vi "CreateSwapArray_v4.vi"(8 "error in (no error)":errorcluster, 9 "ROSCO Params":T3, 11 "ArrayPairs":T1={"iStatus"={"Index"=0, "Value"=0.0}, "TIME"={"Index"=1, "Value"=0.0}, "DT"={"Index"=2, "Value"=0.0}, "BL_PITCH"={"Index"=3, "Value"=0.0}, "VS_MECHGENPWR"={"Index"=13, "Value"=0.0}, "VS_GENPWR"={"Index"=14, "Value"=0.0}, "GEN_SPEED"={"Index"=19, "Value"=0.0}, "ROTOR_SPEED"={"Index"=20, "Value"=0.0}, "GENTQMEAS"={"Index"=22, "Value"=0.0}, "Y_M"={"Index"=23, "Value"=0.0}, "HORWINDV"={"Index"=26, "Value"=0.0}, "ROOTMOOP1"={"Index"=29, "Value"=0.0}, "ROOTMOOP2"={"Index"=30, "Value"=0.0}, "BL_PITCH2"={"Index"=32, "Value"=0.0}, "BL_PITCH3"={"Index"=33, "Value"=0.0}, "ROOTMOOP3"={"Index"=31, "Value"=0.0}, "AVCMSG_SIZE"={"Index"=48, "Value"=0.0}, "INFILE_SIZE "={"Index"=49, "Value"=0.0}, "OUTFILE_SIZE "={"Index"=50, "Value"=0.0}, "FA_ACC"={"Index"=52, "Value"=0.0}, "NUM_BLADES"={"Index"=60, "Value"=0.0}, "OUT_BL_PITCH"={"Index"=44, "Value"=0.0}, "OUT_TORQUE"={"Index"=46, "Value"=0.0}, "OUT_AEROTQ"={"Index"=89, "Value"=0.0}, "Out.RotSpeed "={"Index"=92, "Value"=0.0}, "Out.DEBUG"={"Index"=93, "Value"=0.0}}) -> (0 "error out":errorcluster, 1 "ROSCO Params Out":T3, 3 "ArrayPairs Out":T1={"iStatus"={"Index"=0, "Value"=0.0}, "TIME"={"Index"=1, "Value"=0.0}, "DT"={"Index"=2, "Value"=0.0}, "BL_PITCH"={"Index"=3, "Value"=0.0}, "VS_MECHGENPWR"={"Index"=13, "Value"=0.0}, "VS_GENPWR"={"Index"=14, "Value"=0.0}, "GEN_SPEED"={"Index"=19, "Value"=0.0}, "ROTOR_SPEED"={"Index"=20, "Value"=0.0}, "GENTQMEAS"={"Index"=22, "Value"=0.0}, "Y_M"={"Index"=23, "Value"=0.0}, "HORWINDV"={"Index"=26, "Value"=0.0}, "ROOTMOOP1"={"Index"=29, "Value"=0.0}, "ROOTMOOP2"={"Index"=30, "Value"=0.0}, "BL_PITCH2"={"Index"=32, "Value"=0.0}, "BL_PITCH3"={"Index"=33, "Value"=0.0}, "ROOTMOOP3"={"Index"=31, "Value"=0.0}, "AVCMSG_SIZE"={"Index"=48, "Value"=0.0}, "INFILE_SIZE "={"Index"=49, "Value"=0.0}, "OUTFILE_SIZE "={"Index"=50, "Value"=0.0}, "FA_ACC"={"Index"=52, "Value"=0.0}, "NUM_BLADES"={"Index"=60, "Value"=0.0}, "OUT_BL_PITCH"={"Index"=44, "Value"=0.0}, "OUT_TORQUE"={"Index"=46, "Value"=0.0}, "OUT_AEROTQ"={"Index"=89, "Value"=0.0}, "Out.RotSpeed "={"Index"=92, "Value"=0.0}, "Out.DEBUG"={"Index"=93, "Value"=0.0}}, 4 "avrSWAP":sgl[](array[numeric]))   [LabVIEW 2018]
uses:
  Clusters/RoscoParams.ctl
  Clusters/ArrayPairs.ctl
  Clusters/SwapArrayCluster.ctl
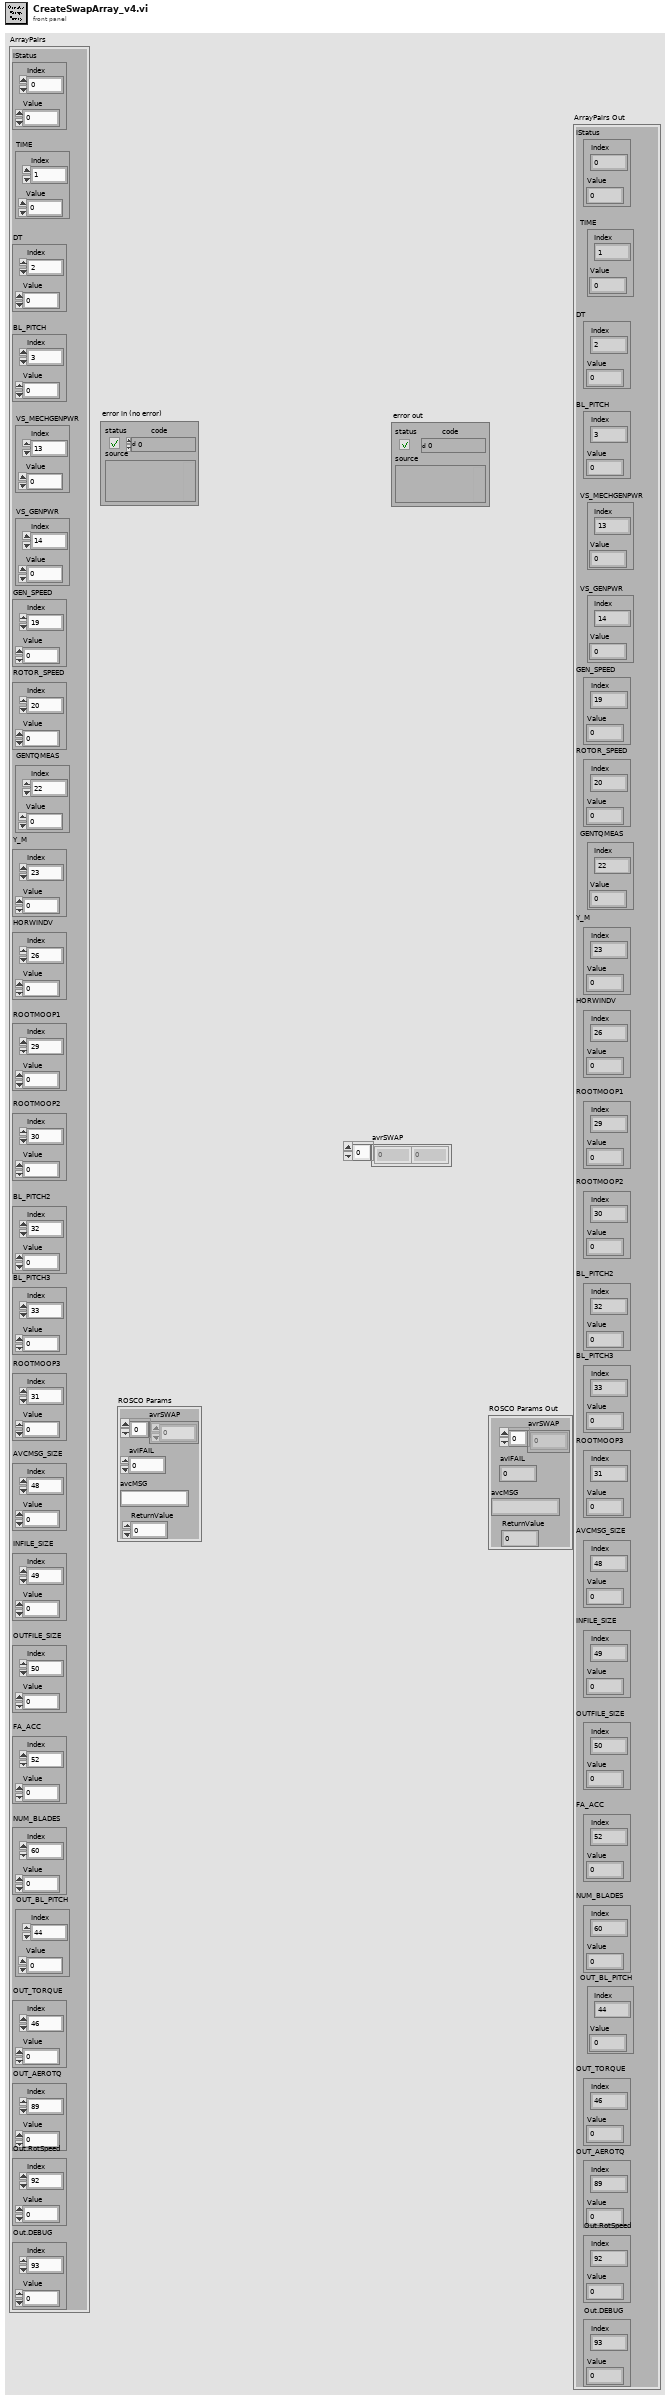
[diagram p1: front panel]
types:
  T1 = typedef "ArrayPairs.ctl" = cluster{"iStatus":T2, "TIME":T2, "DT":T2, "BL_PITCH":T2, "VS_MECHGENPWR":T2, "VS_GENPWR":T2, "GEN_SPEED":T2, "ROTOR_SPEED":T2, "GENTQMEAS":T2, "Y_M":T2, "HORWINDV":T2, "ROOTMOOP1":T2, "ROOTMOOP2":T2, "BL_PITCH2":T2, "BL_PITCH3":T2, "ROOTMOOP3":T2, "AVCMSG_SIZE":T2, "INFILE_SIZE ":T2, "OUTFILE_SIZE ":T2, "FA_ACC":T2, "NUM_BLADES":T2, "OUT_BL_PITCH":T2, "OUT_TORQUE":T2, "OUT_AEROTQ":T2, "Out.RotSpeed ":T2, "Out.DEBUG":T2}
  T2 = typedef "SwapArrayCluster.ctl" = cluster{"Index":i32, "Value":dbl}
  T3 = typedef "RoscoParams.ctl" = cluster{"avrSWAP":sgl[], "aviFAIL":i32, "avcMSG":string, "ReturnValue":i32}
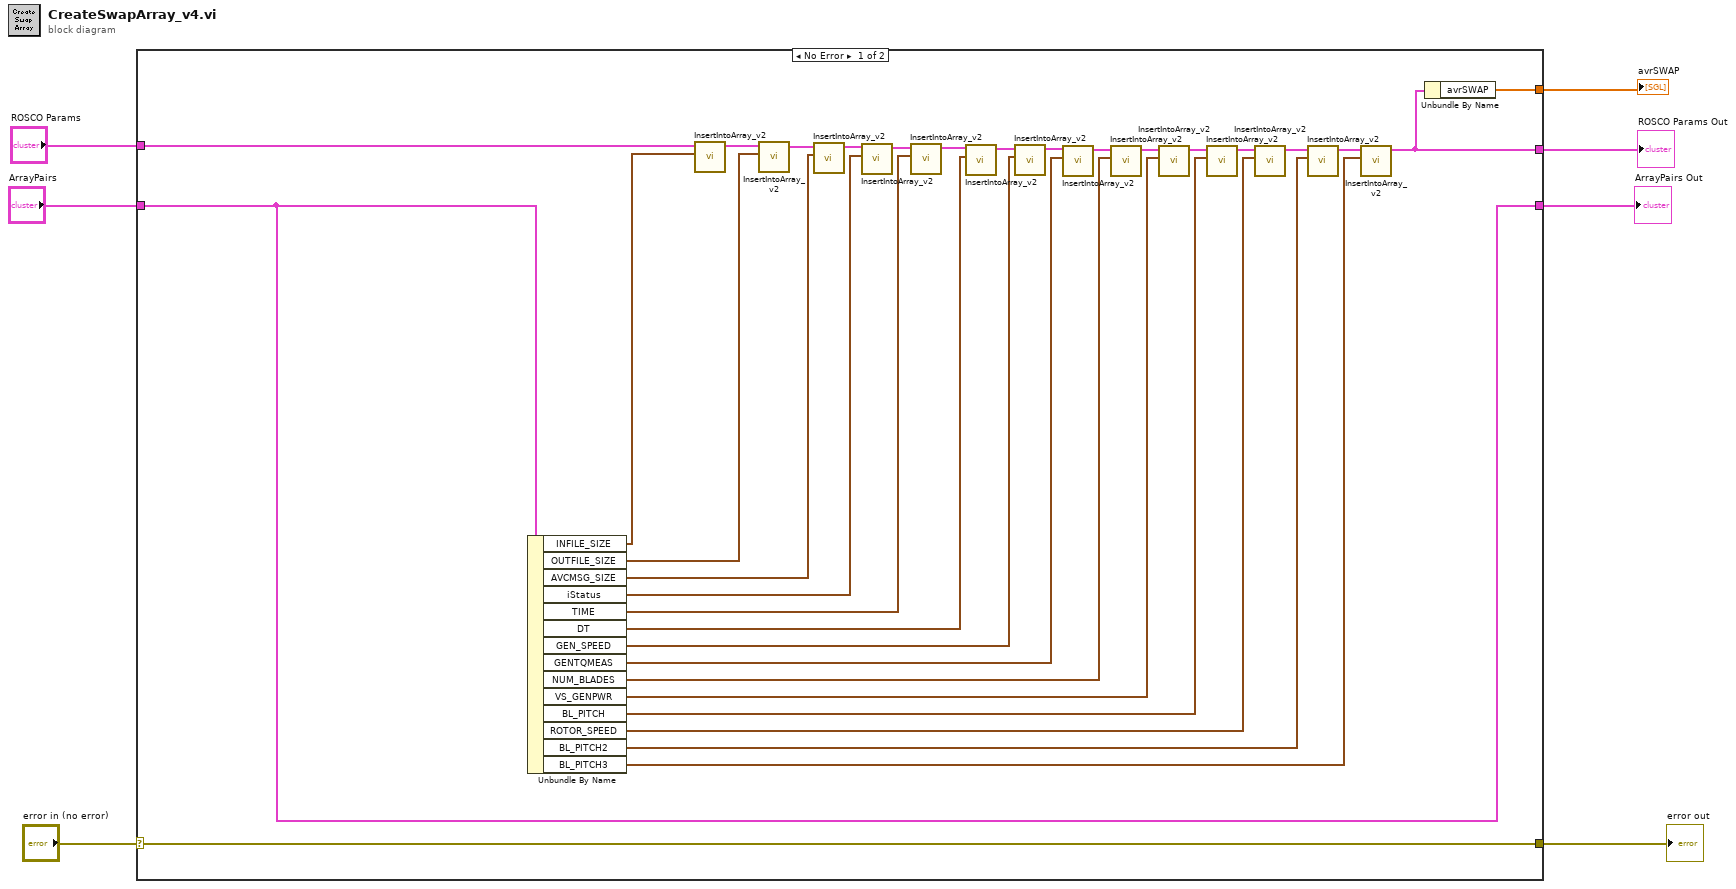
[diagram p0: block diagram]
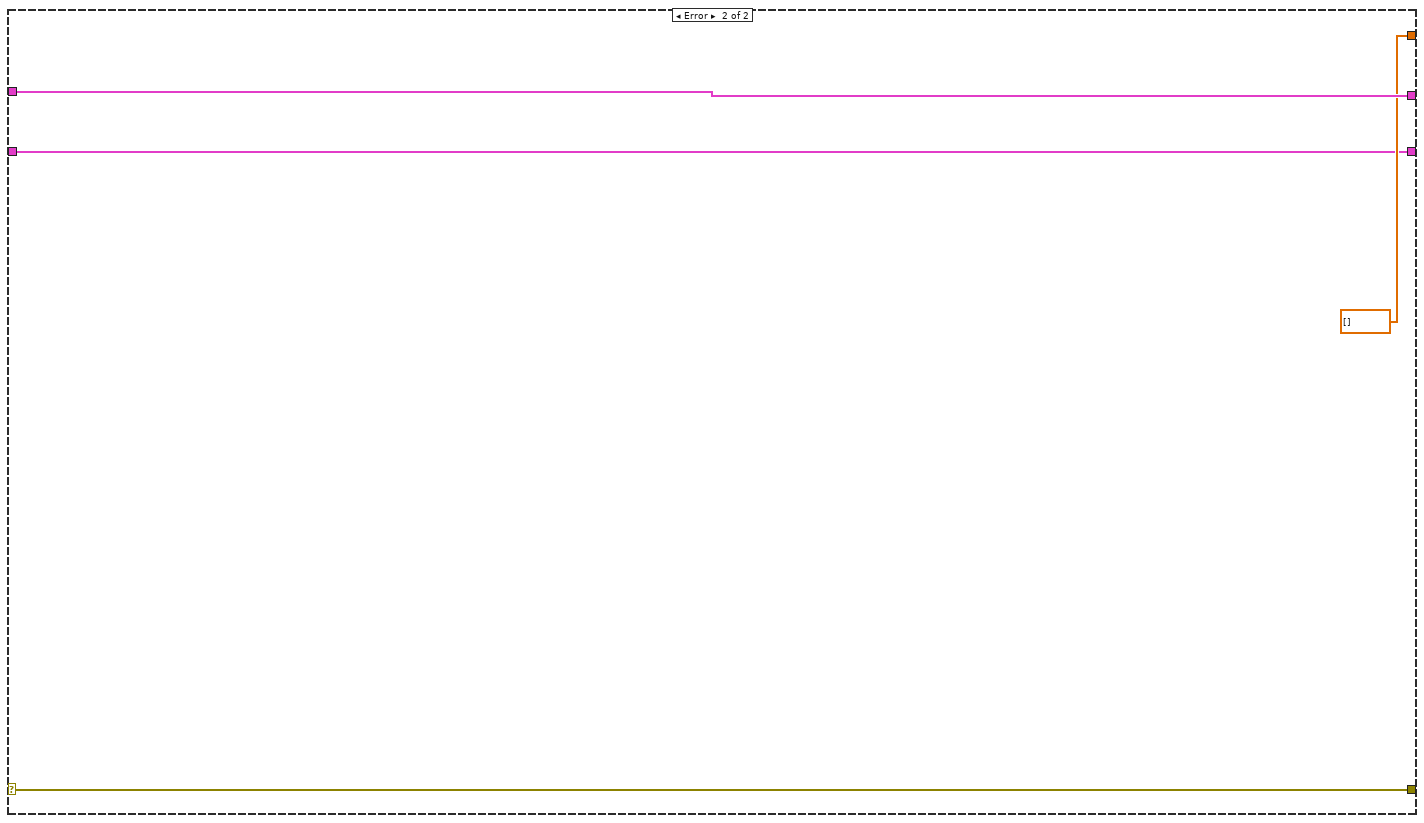
[diagram p2: hidden frame]
diagram:
  n1 = case shown="No Error" "error in (no error)" {
    selector: "error in (no error)" -> [w12 w42]
    tunnel: "ROSCO Params" -> [w39 w43]
    tunnel: [w8 w43] -> w6
    tunnel: "ArrayPairs" -> [w9 w40]
    tunnel: [w12 w42] -> w4
    tunnel: [w13 sgl[] [] ("avrSWAP")] -> w2
    tunnel: [w9 w40] -> w1
    frame No Error {
      n2 = Unbundle By Name(w9) -> ("INFILE_SIZE"=w38:T2, "OUTFILE_SIZE"=w32:T2, "AVCMSG_SIZE"=w30:T2, "iStatus"=w29:T2, "TIME"=w28:T2, "DT"=w21:T2, "GEN_SPEED"=w20:T2, "GENTQMEAS"=w19:T2, "NUM_BLADES"=w18:T2, "VS_GENPWR"=w17:T2, "BL_PITCH"=w16:T2, "ROTOR_SPEED"=w15:T2, "BL_PITCH2"=w14:T2, "BL_PITCH3"=w11:T2)
      n3 = call "InsertIntoArray_v2.vi"("ROSCO Params"=w39, "KeyVal"=w38) -> ("ROSCO Params Out"=w37:T3)  [unwired: 7 in, 1 out]
      n4 = call "InsertIntoArray_v2.vi"("ROSCO Params"=w37, "KeyVal"=w32) -> ("ROSCO Params Out"=w31:T3)  [unwired: 7 in, 1 out]
      n5 = call "InsertIntoArray_v2.vi"("ROSCO Params"=w31, "KeyVal"=w30) -> ("ROSCO Params Out"=w27:T3)  [unwired: 7 in, 1 out]
      n6 = call "InsertIntoArray_v2.vi"("ROSCO Params"=w27, "KeyVal"=w29) -> ("ROSCO Params Out"=w36:T3)  [unwired: 7 in, 1 out]
      n7 = call "InsertIntoArray_v2.vi"("ROSCO Params"=w36, "KeyVal"=w28) -> ("ROSCO Params Out"=w26:T3)  [unwired: 7 in, 1 out]
      n8 = call "InsertIntoArray_v2.vi"("ROSCO Params"=w26, "KeyVal"=w21) -> ("ROSCO Params Out"=w35:T3)  [unwired: 7 in, 1 out]
      n9 = call "InsertIntoArray_v2.vi"("ROSCO Params"=w35, "KeyVal"=w20) -> ("ROSCO Params Out"=w25:T3)  [unwired: 7 in, 1 out]
      n10 = call "InsertIntoArray_v2.vi"("ROSCO Params"=w25, "KeyVal"=w19) -> ("ROSCO Params Out"=w34:T3)  [unwired: 7 in, 1 out]
      n11 = call "InsertIntoArray_v2.vi"("ROSCO Params"=w34, "KeyVal"=w18) -> ("ROSCO Params Out"=w24:T3)  [unwired: 7 in, 1 out]
      n12 = call "InsertIntoArray_v2.vi"("ROSCO Params"=w24, "KeyVal"=w17) -> ("ROSCO Params Out"=w23:T3)  [unwired: 7 in, 1 out]
      n13 = call "InsertIntoArray_v2.vi"("ROSCO Params"=w23, "KeyVal"=w16) -> ("ROSCO Params Out"=w33:T3)  [unwired: 7 in, 1 out]
      n14 = call "InsertIntoArray_v2.vi"("ROSCO Params"=w33, "KeyVal"=w15) -> ("ROSCO Params Out"=w22:T3)  [unwired: 7 in, 1 out]
      n15 = call "InsertIntoArray_v2.vi"("ROSCO Params"=w22, "KeyVal"=w14) -> ("ROSCO Params Out"=w10:T3)  [unwired: 7 in, 1 out]
      n16 = call "InsertIntoArray_v2.vi"("ROSCO Params"=w10, "KeyVal"=w11) -> ("ROSCO Params Out"=w8:T3)  [unwired: 7 in, 1 out]
      n17 = Unbundle By Name(w8) -> ("avrSWAP"=w13:sgl[])
    }
    frame Error {
    }
  }
  "error out" <- w4
  "ROSCO Params Out" <- w6
  "avrSWAP" <- w2
  "ArrayPairs Out" <- w1
